vi "Read Max Pressure Released.vi"(11 "Volcano in":refnum<class "Volcano.lvclass">) -> (2 "Max Pressure Released":u64, 3 "Volcano out":refnum<class "Volcano.lvclass">)   [LabVIEW 2021, in "d16.lvlib" / "Volcano.lvclass"]
uses:
  Volcano.lvclass
  Volcano.lvclass/Volcano.ctl
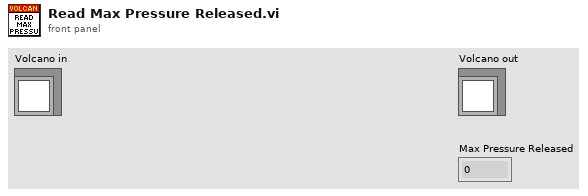
[diagram p1: front panel]
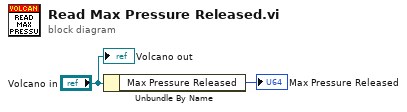
[diagram p0: block diagram]
diagram:
  n1 = Unbundle By Name("Volcano in") -> ("Max Pressure Released"=→"Max Pressure Released":u64)
  "Volcano out" <- "Volcano in"
